vi "Q8381 REF LEVEL_REF LEVEL.vi"(1 "unit":u16(ring) items=["dBm ", "mW", "uW", "nW"], 2 "value":dbl format="%.1f", 3 "GPIB Address":u16=8 max=31 step=1, 4 "VISA resource name":refnum<visa-resource-name>) -> (0 "GPIB Status":bool)   [LabVIEW 2017]
doc: "unit: 0: dBm, 1: mW, 2: uW, 3: nW"
panel:
  out "Program Code":string
  # "REF  LEVEL__REF  LEVEL"
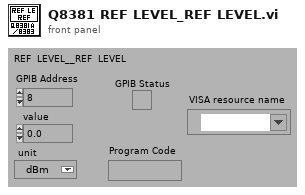
[diagram p1: front panel]
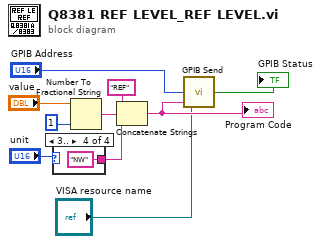
[diagram p0: block diagram]
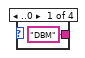
[diagram p2: hidden frame]
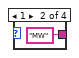
[diagram p3: hidden frame]
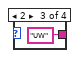
[diagram p4: hidden frame]
diagram:
  n1 = case shown="3.." "unit" {
    tunnel: ["DBM" "MW" "UW" "NW"] -> w5
    frame ..0 {
    }
    frame 1 {
    }
    frame 2 {
    }
    frame 3.. {
    }
  }
  n2 = Number To Fractional String(number="value", precision (6)=1) -> (F-format string=w9:string)  [unwired: 2 in]
  n3 = Concatenate Strings("REF", w9, w5) -> (w4:string)
  "Program Code" <- w4
  n4 = call "GPIB Send.vi"("Command String"=w4, "Address"="GPIB Address", "VISA resource name"="VISA resource name") -> ("Error"=→"GPIB Status":bool)
